vi "U32 to Data Type.vi"(8 "error in (no error)":errorcluster, 11 "U32":u32) -> (0 "error out":errorcluster, 3 "Boolean out":refnum<class "U32.lvclass">)   [LabVIEW 2017, in "U32.lvclass"]
uses:
  <vilib>/gpm_packages/@cs/data-type-serializer/source/U32/U32.lvclass
  <vilib>/gpm_packages/@cs/data-type-serializer/source/U32/U32.lvclass/U32.ctl
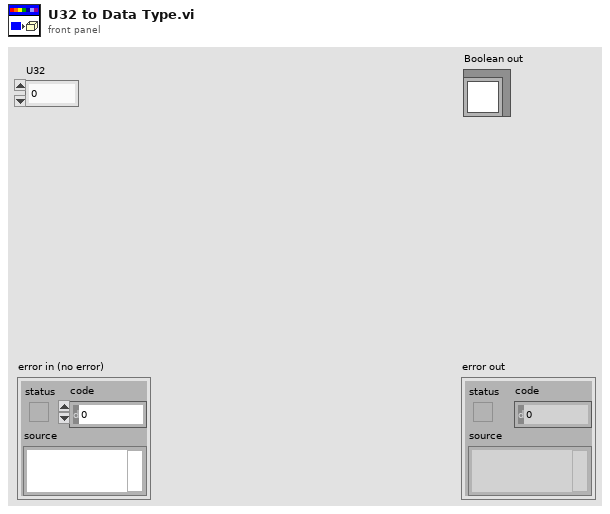
[diagram p1: front panel]
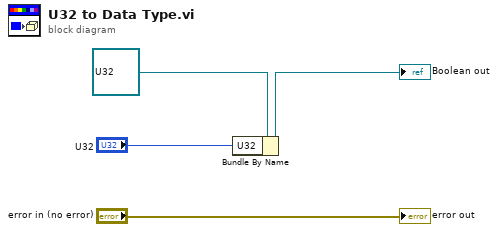
[diagram p0: block diagram]
diagram:
  n1 = Bundle By Name(cluster=refnum<class "U32.lvclass"> refnum ("Boolean in"), "U32"="U32") -> (→"Boolean out":refnum<class "U32.lvclass">)
  "error out" <- "error in (no error)"
